vi "SimpleSerialCom.vi"() -> ()   [LabVIEW 2017]
panel:
  in  "Radio Buttons":T1(radio)
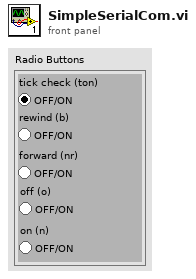
[diagram p1: front panel]
types:
  T1 = enum32{"tick check (ton)", "rewind (b)", "forward (nr)", "off (o)", "on (n)"}
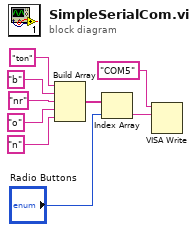
[diagram p0: block diagram]
diagram:
  n1 = Build Array("ton", "b", "nr", "o", "n") -> (w5:string[])
  n2 = Index Array(array=w5, index="Radio Buttons") -> (element=w3:string)
  n3 = VISA Write(VISA resource name="COM5", write buffer=w3) -> ()  [unwired: 1 in, 3 out]
